vi "Tab.vi"(4 "Time Stamp":timestamp=timestamp(3382702114 s since 1904-01-01), 6 "String":string="FooBar", 8 "Array":path[](array[path])=[path "\\\\nirvana\\temp/jah/DefaultValues/Enums.vi"], 9 "Real Matrix":dbl[][](array[numeric])=[[1.0, 2.0, 3.0], [4.0, 5.0, 6.0]], 10 "Numeric":u32=123, 11 "Options (Tab Control)":T1(tab)) -> ()   [LabVIEW 2011]
panel:
  in  "stop":bool
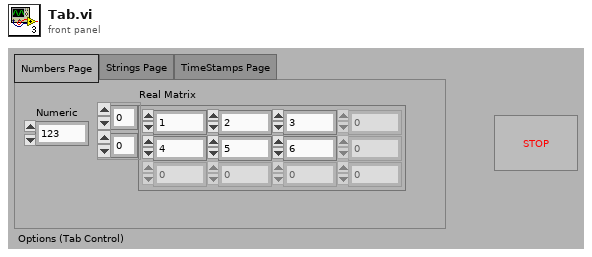
[diagram p1: front panel]
types:
  T1 = enum32{"Numbers Page", "Strings Page", "TimeStamps Page"}
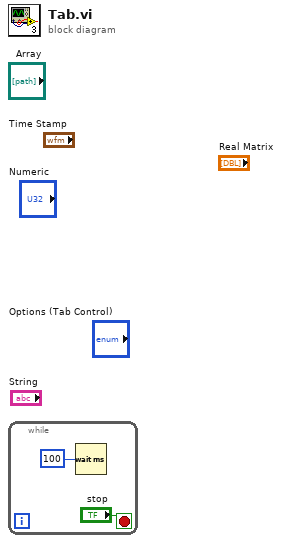
[diagram p0: block diagram]
diagram:
  n1 = while {
    stop <- "stop" stop-if-true
    n2 = Wait (ms)(milliseconds to wait=u32 100) -> ()  [unwired: 1 out]
  }
